vi "poly_range_I32.vi"(8 "inclusive (T)":bool=TRUE, 9 "end":i32, 10 "beginning":i32) -> (1 "range":i32[](array[numeric]), 2 "N":i32)   [LabVIEW 2015]
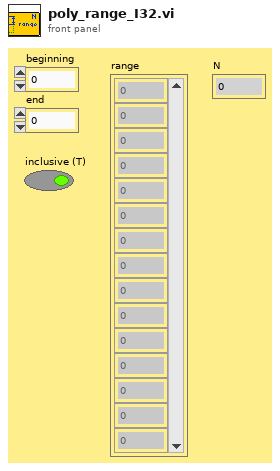
[diagram p1: front panel]
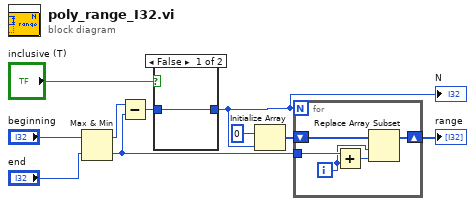
[diagram p0: block diagram]
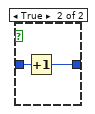
[diagram p2: hidden frame]
diagram:
  n1 = Max & Min(x="beginning", y="end") -> (max(x,y)=w8:i32, min(x,y)=w5:i32)
  n2 = Subtract(x=w8, y=w5) -> (x-y=w3:i32)
  n3 = case shown="False" "inclusive (T)" {
    tunnel: w3 -> [w11 w13]
    tunnel: [w11 w12] -> w2
    frame False {
    }
    frame True {
      n4 = Increment(x=w13) -> (x+1=w12:i32)
    }
  }
  "N" <- w2
  n5 = Initialize Array(0, w2) -> (w6:i32[])
  n6 = for {
    N: w2 -> [_]
    shift-right: [w14] -> w4
    shift-left: w6 -> [w18]
    tunnel: w5 -> [w17]
    i -> [w16]
    n7 = Add(x=w17, y=w16) -> (x+y=w15:i32)
    n8 = Replace Array Subset(array=w18, new element=w15, index=w16) -> (w14:i32[])
  }
  "range" <- w4
